vi "Set Current Ramp Rate_brasse.vi"(0 "Communications Config":T1={"GPIB address"=22, "GPIB bus"=0, "connection ID"=refnum, "IP"="192.168.2.200", "Active Comm Interface"=0, "Serial Port"="", "Programmer Type"=0} {"Programmer Type" items=["Model 430", "Model 420"]; "Active Comm Interface" items=["TCP/IP (Model 430 Only)", "RS232", "IEEE488"]}, 1 "Segment":i32=1, 2 "Ramp Rate (A/sec)":dbl format="%.5f", 3 "error in":T2, 4 "Upper Bounds":dbl=40.0) -> (5 "error out":T2)   [LabVIEW 2009]
panel:
  out "output string":string
  in  "GPIB Address":cluster{"GPIB address":i16, "GPIB bus":i16}={"GPIB address"=22, "GPIB bus"=0}
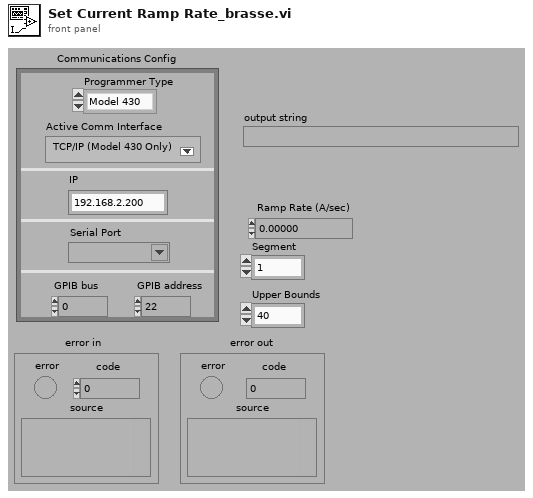
[diagram p1: front panel]
types:
  T1 = cluster{"GPIB address":i16, "GPIB bus":i16, "connection ID":refnum<k5>, "IP":string, "Active Comm Interface":u16, "Serial Port":refnum<visa-resource-name>, "Programmer Type":u16}
  T2 = cluster{"error":bool, "code":i32, "source":string}
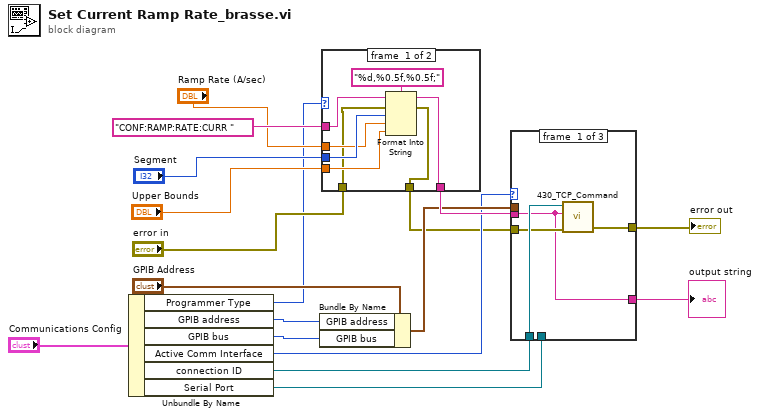
[diagram p0: block diagram]
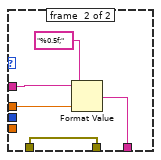
[diagram p2: hidden frame]
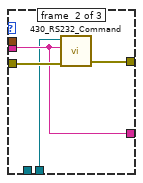
[diagram p3: hidden frame]
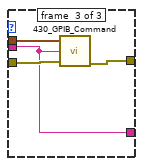
[diagram p4: hidden frame]
diagram:
  n1 = Unbundle By Name("Communications Config") -> ("Programmer Type"=w1:u16, "GPIB address"=w12:i16, "GPIB bus"=w11:i16, "Active Comm Interface"=w7:u16, "connection ID"=w10:refnum<k5>, "Serial Port"=w3:refnum<visa-resource-name>)
  n2 = Bundle By Name(cluster="GPIB Address", "GPIB address"=w12, "GPIB bus"=w11) -> (w13:cluster{"GPIB address":i16, "GPIB bus":i16})
  n3 = case shown="1" w1 {
    tunnel: "CONF:RAMP:RATE:CURR " -> [w26 w31]
    tunnel: "Ramp Rate (A/sec)" -> [w24 w30]
    tunnel: [w22 w28] -> w16
    tunnel: "Segment" -> [w25 _]
    tunnel: "Upper Bounds" -> [w23 _]
    tunnel: "error in" -> [w21 w27]
    tunnel: [w20 w27] -> w5
    frame #0 {
      n4 = Format Into String(format string="%d,%0.5f,%0.5f;", initial string=w26, error in=w21, w25, w24, w23) -> (resulting string=w22:string, error out=w20:errorcluster)
    }
    frame #1 {
      n5 = Format Value(string ("")=w31, format string="%0.5f;", value (0)=w30) -> (output string=w28:string)
    }
  }
  n6 = case shown="2" w7 {
    tunnel: w16 -> [w32 w37 w40]
    tunnel: w5 -> [w34 w39 w43]
    tunnel: [w33 w38 w42] -> w15
    tunnel: w13 -> [_ _ w41]
    tunnel: w10 -> [w35 _ _]
    tunnel: [w32 w37 w40] -> w4
    tunnel: w3 -> [_ w36 _]
    frame #0 {
      n7 = call <userlib>:"430_TCP_Command.vi"("error in (no error)"=w34, "Command"=w32, "connection ID"=w35) -> ("error out"=w33:errorcluster)  [unwired: 1 in, 2 out]
    }
    frame #1 {
      n8 = call <userlib>:"430_RS232_Command.vi"("error in (no error)"=w39, "Command"=w37, "VISA resource name"=w36) -> ("error out"=w38:errorcluster)  [unwired: 1 in, 2 out]
    }
    frame #2 {
      n9 = call <userlib>:"430_GPIB_Command.vi"("GPIB (In)"=w41, "Input command"=w40, "error in"=w43) -> ("error out"=w42:T2)  [unwired: 3 out]
    }
  }
  "error out" <- w15
  "output string" <- w4
